vi "Write Subdiagram Label.vi"(8 "Error In":errorcluster) -> (0 "Error Out":errorcluster)   [LabVIEW 2018, in "Tests.lvlib" / "Toolkit.lvlib"]
uses:
  Toolkit.lvlib
  <vilib>/Utility/traverseref.llb/TRef TravTarget.ctl
  <vilib>/addons/_JKI Toolkits/Caraya/classes/Test/Test.lvclass
  src/Toolkit/Toolkit.lvlib
  <vilib>/Utility/traverseref.llb/VI Scripting - Traverse.lvlib
  <vilib>/addons/_JKI Toolkits/Caraya/classes/Assert/Assert.lvclass
  Tests.lvlib
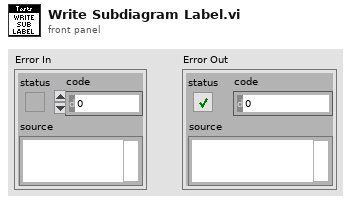
[diagram p1: front panel]
types:
  T1 = typedef "TRef TravTarget.ctl" = enum16{"FP", "BD", "Other"}
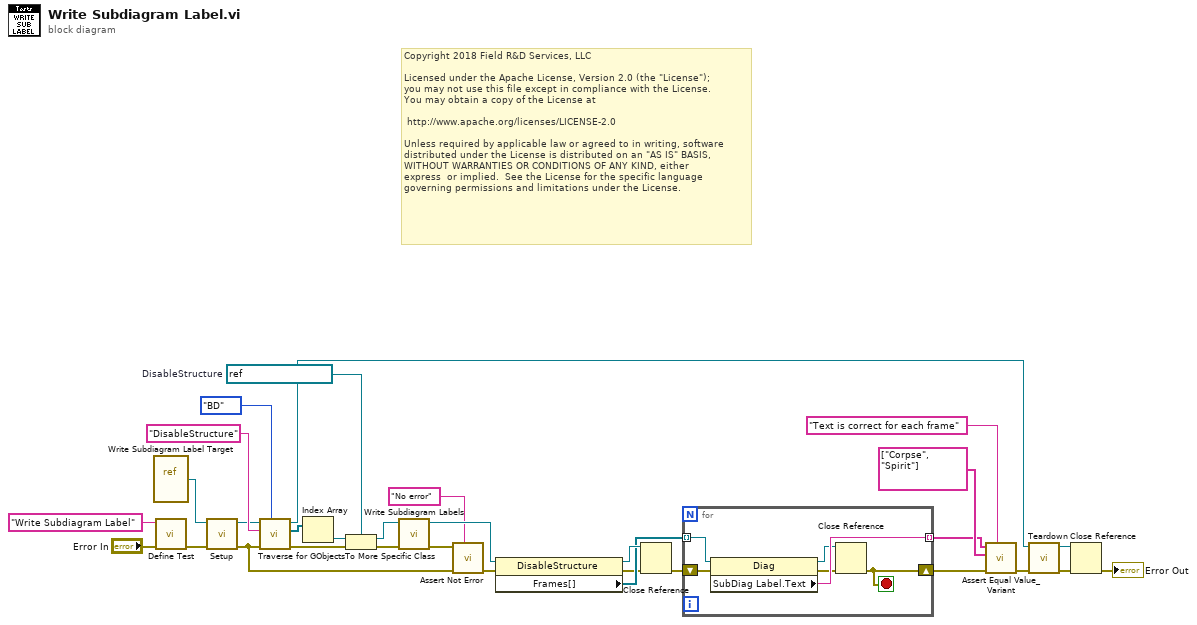
[diagram p0: block diagram]
diagram:
  w25 = refnum<vi> refnum  # DisableStructure
  # "Copyright 2018 Field R&D Services, LLC\n\nLicensed under the Apache License, Version 2.0 (the \"License\");\nyou may not use this file except in compliance with the License.\nYou may obtain a copy of the License at\n\n\thttp://www.apache.org/licenses/LICENSE-2.0\n\nUnless required by applicable law or agreed to in writing, software\ndistributed under the License is distributed on an \"AS IS\" BASIS,\nWITHOUT WARRANTIES OR CONDITIONS OF ANY KIND, either \nexpress  or implied.  See the License for the specific language \ngoverning permissions and limitations under the License."
  n1 = vi-ref "Write Subdiagram Label Target.vi"() -> (w23:refnum<vi>)
  n2 = call <vilib>:"Define Test.vi"("error in (no error)"="Error In", "Label (VI Title)"="Write Subdiagram Label") -> ("error out"=w14:errorcluster)  [unwired: 9 in]
  n3 = call "Setup.vi"("Error In"=w14, "VI In"=w23) -> ("Error Out"=w6:errorcluster, "VI Out"=w22:refnum<vi>)  [unwired: 8 in]
  n4 = call <vilib>:"Traverse for GObjects.vi"("Traverse Target"=TRef_TravTarget."BD", "error in (no error)"=w6, "Class Name"="DisableStructure", "VI Refnum"=w22) -> ("error out"=w28:errorcluster, "References"=w27:refnum<vi>[], "dup VI Refnum"=w21:refnum<vi>)  [unwired: 4 in, 1 out]
  n5 = Index Array(array=w27) -> (element=w26:refnum<vi>)  [unwired: 1 in]
  n6 = To More Specific Class(target class=w25, reference=w26, error in=w28) -> (specific class reference=w24:refnum<vi>, error out=w7:errorcluster)
  n7 = call "Write Subdiagram Labels.vi"("Error In"=w7, "DisableStructure In"=w24) -> ("Error Out"=w3:errorcluster, "DisableStructure Out"=w17:refnum<vi>)  [unwired: 8 in]
  n8 = call <vilib>:"Assert Not Error.vi"("Label"="No error", "error in (no error)"=w6, "Not Error?"=w3) -> ("error out"=w5:errorcluster)  [unwired: 8 in]
  n9 = property class="DisableStructure"(reference=w17, error in=w5) -> (reference out=w16:refnum<vi>, error out=w13:errorcluster, "Frames[]"=w15:refnum<vi>[])
  n10 = Close Reference(reference=w16, error in (no error)=w13) -> (error out=w12:errorcluster)
  n11 = for {
    tunnel: w15 -> [w37] mode=indexing
    tunnel: [w35] -> w10 mode=indexing
    shift-right: [w33] -> w4
    shift-left: w12 -> [w36]
    stop <- w33 stop-if-true
    n12 = property class="Diag"(reference=w37, error in=w36) -> (reference out=w32:refnum<vi>, error out=w34:errorcluster, "SubDiag Label.Text"=w35:string)
    n13 = Close Reference(reference=w32, error in (no error)=w34) -> (error out=w33:errorcluster)
  }
  n14 = call <vilib>:"Assert Equal Value_Variant.vi"("Label"="Text is correct for each frame", "error in (no error)"=w4, "Y"=string[] ["Corpse", "Spirit"], "X"=w10) -> ("error out"=w8:errorcluster)  [unwired: 7 in]
  n15 = call "Teardown.vi"("Error In"=w8, "VI In"=w21) -> ("Error Out"=w19:errorcluster, "VI Out"=w20:refnum<vi>)  [unwired: 8 in]
  n16 = Close Reference(reference=w20, error in (no error)=w19) -> (error out=→"Error Out":errorcluster)
